vi "Loop Set Bleed-Fuel-ECS Cntrls.vi"(8 "error in (no error)":errorcluster, 11 "Bleed-Fuel-ECS Controls":T1 {"Bleed-Coarse-Knob" min=4.0 max=20.0 step=0.001 scale=4.0..20.0; "Bleed-Fine-Knob" min=4.0 max=20.0 step=0.001 scale=4.0..20.0}) -> (0 "error out":errorcluster)   [LabVIEW 2018]
doc: "This subVI enqueues the named action in to the communications queue along with the input data."
uses:
  Private Controls/Module Action.ctl
  RT - Instrument IO.lvlib
  Private Controls/Module Data.ctl
  Modules/Testing UI 1/Public Controls/Bleed-Fuel-ECS Controls.ctl
  Modules/Testing UI 1/Testing UI 1.lvlib
panel:
  # "Bleed Load Controls"
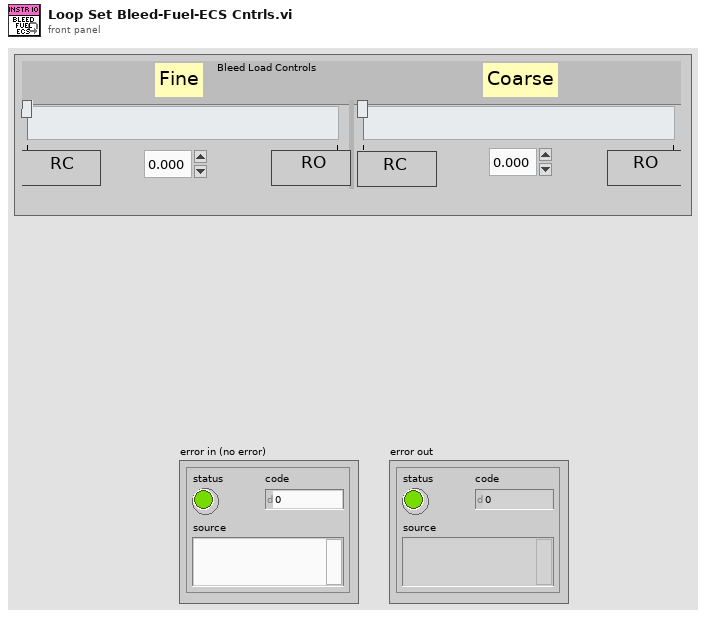
[diagram p1: front panel]
types:
  T1 = typedef "Testing UI 1.lvlib/Bleed-Fuel-ECS Controls.ctl" = cluster{"Fine_RC":bool, "Fine_RO":bool, "Coarse_RC":bool, "Coarse_RO":bool, "Bleed-Fine-Knob":dbl, "Bleed-Coarse-Knob":dbl}
  T2 = typedef "RT - Instrument IO.lvlib/Module Data.ctl" = cluster{"Data":variant, "Action":T3}
  T3 = typedef "RT - Instrument IO.lvlib/Module Action.ctl" = enum16{"Init", "Error", "StartStop Acquisition", "Write 02-06-9265 Vals (AO)", "Write 00-04-9265 Vals (AO)", "Write 02-00-9485 Vals (DO)", "Write 02-01-9485 Vals (DO)", "Set APU&ECU Cntrls", "Set Bleed-Fuel-ECS Cntrls", "Loop Set Bleed-Fuel-ECS Cntrls", "Set ECS Demnd Cluster", "Set Fuel Pres Regltr", "Set Overspeed Thresholds", "Write Single 02-00-9485 Chann", "Write Single 02-01-9485 Chann", "Write Single 00-04-9265 Chann", "Set Sample Rate", "ESTOP"}
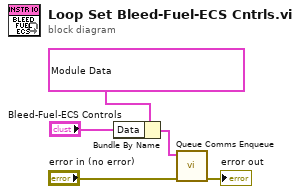
[diagram p0: block diagram]
diagram:
  n1 = Bundle By Name(cluster=T2 {"Data"=variant, "Action"=enum."Loop Set Bleed-Fuel-ECS Cntrls"} ("element"), "Data"="Bleed-Fuel-ECS Controls") -> (w5:T2)
  n2 = call "Queue Comms Enqueue.vi"("error in (no error)"="error in (no error)", "element"=w5) -> ("error out"=→"error out":errorcluster)  [unwired: 9 in]
